vi "Read Write VI example.vi"(0 "GEA2 Reference In":refnum<k24>, 5 "Board Index":i32, 7 "GEA Inputs":T5={"Source"=228, "Destination"=35} {"Destination" format="%.0x"; "Source" format="%.0x"}, 9 "Stand Alone?":bool=TRUE, 11 "error in":errorcluster) -> (4 "GEA2 Reference Out":refnum<k24>, 6 "ERD Read Out":T4[](array[typedef]) {"ERD Number" format="%.0x"}, 15 "error out":errorcluster)   [LabVIEW 2016]
uses:
  Common/LabVIEW GEA2 Toolkit/LabVIEW_GEA2_Toolkit.lvlibp/type defs/Source_Destination.ctl
  Q:/Common/DLLs/GEA3/GeaCommunication.dll
  Common/DLLs/GEA3/GeaCommunication.dll
  Common/LabVIEW GEA2 Toolkit/LabVIEW_GEA2_Toolkit.lvlibp/type defs/ERD Read Data Out.ctl
  Common/LabVIEW GEA2 Toolkit/LabVIEW_GEA2_Toolkit.lvlibp/type defs/ERD Write Data In.ctl
  Common/LabVIEW GEA2 Toolkit/LabVIEW_GEA2_Toolkit.lvlibp/type defs/Data Type.ctl
  Common/LabVIEW GEA2 Toolkit/LabVIEW_GEA2_Toolkit.lvlibp/type defs/ERD Read Data In.ctl
  Common/LabVIEW GEA2 Toolkit/LabVIEW_GEA2_Toolkit.lvlibp
panel:
  out "ERD Write out":string
  in  "ERD Read Data In":T1 {"ERD Number" format="%.0x"}
  in  "ERD Write Data In":T3={"ERD Number"=0, "Data Type"=enum."string", "Data"="0"} {"ERD Number" format="%.0x"}
  in  "Read ERD":bool
  in  "Write ERD":bool
  in  "Stop Button":bool
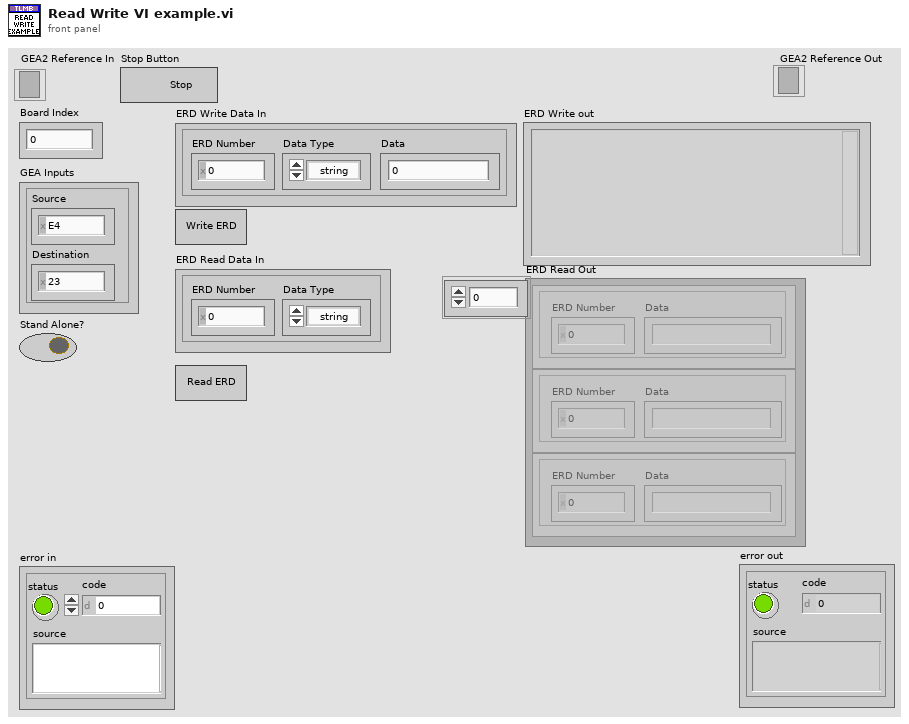
[diagram p1: front panel]
types:
  T1 = typedef "LabVIEW_GEA2_Toolkit.lvlibp/ERD Read Data In.ctl" = cluster{"ERD Number":u16, "Data Type":T2}
  T2 = typedef "LabVIEW_GEA2_Toolkit.lvlibp/Data Type.ctl" = enum16{"string", "boolean", "uint8_t", "uint16_t", "uint32_t", "uint64_t", "int8_t", "int16_t", "int32_t", "int64_t"}
  T3 = typedef "LabVIEW_GEA2_Toolkit.lvlibp/ERD Write Data In.ctl" = cluster{"ERD Number":u16, "Data Type":T2, "Data":string}
  T4 = typedef "LabVIEW_GEA2_Toolkit.lvlibp/ERD Read Data Out.ctl" = cluster{"ERD Number":u16, "Data":string}
  T5 = typedef "LabVIEW_GEA2_Toolkit.lvlibp/Source_Destination.ctl" = cluster{"Source":u8, "Destination":u8}
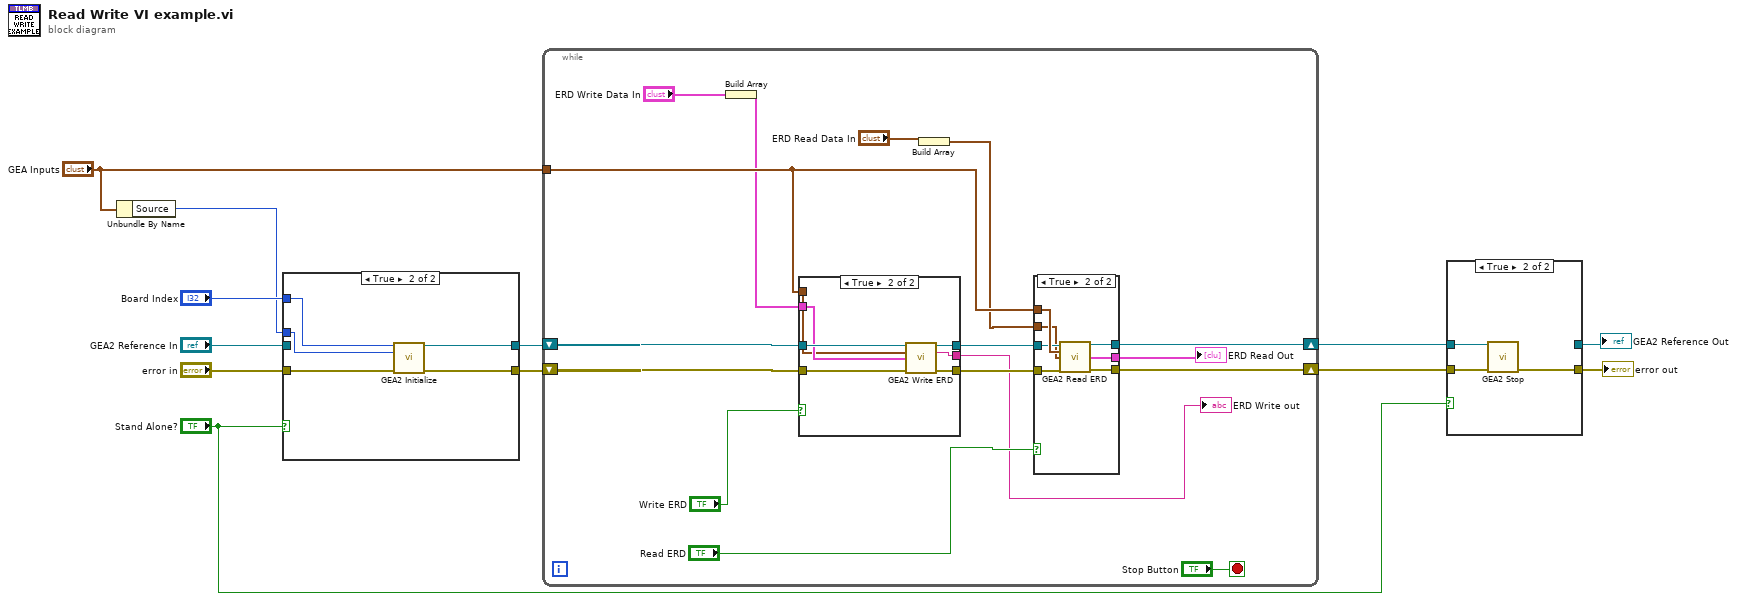
[diagram p0: block diagram]
diagram:
  n1 = Unbundle By Name("GEA Inputs") -> ("Source"=w10:u8)
  n2 = case shown="True" "Stand Alone?" {
    tunnel: "Board Index" -> [_ w19]
    tunnel: w10 -> [_ w18]
    tunnel: "error in" -> [w13 w17]
    tunnel: [w14 w16] -> w8
    tunnel: [w13 w15] -> w7
    tunnel: "GEA2 Reference In" -> [w14 _]
    frame False {
    }
    frame True {
      n3 = call "GEA2 Initialize.vi"("Board Index"=w19, "Source Address"=w18, "error in"=w17) -> ("GEA2 Reference Out"=w16:refnum<k24>, "error out"=w15:errorcluster)  [unwired: 10 in, 1 out]
    }
  }
  n4 = while {
    tunnel: "GEA Inputs" -> [w33]
    shift-right: [w30] -> w5
    shift-left: w8 -> [w35]
    shift-right: [w29] -> w4
    shift-left: w7 -> [w34]
    stop <- "Stop Button" stop-if-true
    n5 = Build Array("ERD Write Data In") -> (w23:T3[])
    n6 = case shown="True" "Write ERD" {
      tunnel: w35 -> [w46 w53]
      tunnel: w34 -> [w45 w52]
      tunnel: w23 -> [_ w51]
      tunnel: w33 -> [_ w50]
      tunnel: [w46 w49] -> w32
      tunnel: [w45 w48] -> w31
      tunnel: [_ w47] -> w20
      frame False {
      }
      frame True {
        n7 = call "GEA2 Write ERD.vi"("GEA2 Reference In"=w53, "GEA Inputs"=w50, "Write ERD List"=w51, "Error In"=w52) -> ("GEA2 Reference Out"=w49:refnum<k24>, "Raw Data Out"=w47:string, "Error Out"=w48:errorcluster)  [unwired: 9 in]
      }
    }
    "ERD Write out" <- w20
    n8 = Build Array("ERD Read Data In") -> (w21:T1[])
    n9 = case shown="True" "Read ERD" {
      tunnel: w33 -> [_ w44]
      tunnel: w32 -> [w37 w43]
      tunnel: w31 -> [w36 w42]
      tunnel: [w37 w41] -> w30
      tunnel: [w36 w40] -> w29
      tunnel: [_ w39] -> w25
      tunnel: w21 -> [_ w38]
      frame False {
      }
      frame True {
        n10 = call "GEA2 Read ERD.vi"("GEA2 Reference In"=w43, "GEA Inputs"=w44, "Read ERD List"=w38, "Error In"=w42) -> ("GEA2 Reference Out"=w41:refnum<k24>, "ERD Data Out"=w39:T4[], "Error Out"=w40:errorcluster)  [unwired: 8 in, 1 out]
      }
    }
    "ERD Read Out" <- w25
  }
  n11 = case shown="True" "Stand Alone?" {
    tunnel: w5 -> [w55 w58]
    tunnel: w4 -> [w54 w57]
    tunnel: [w54 w56] -> w3
    tunnel: [w55 _] -> w2
    frame False {
    }
    frame True {
      n12 = call "GEA2 Stop.vi"("GEA2 Reference In"=w58, "Error In"=w57) -> ("Error Out"=w56:errorcluster)  [unwired: 13 in]
    }
  }
  "GEA2 Reference Out" <- w2
  "error out" <- w3
